vi "翻译助手.vi"() -> ()   [LabVIEW 2014]
uses:
  <vilib>/httpClient/LabVIEWHTTPClient.lvlib
  <vilib>/addons/JSON API/JSON Value/JSON Value.lvclass
  <vilib>/addons/JSON API/JSON Scalar/JSON Scalar.lvclass
panel:
  in  "确定按钮":bool
  in  "目标语言":u16(ring) items=["自动检测", "中文", "英文", "日文", "俄文", "文言文", "粤语", "繁体中文"]
  in  "源语言":u16(ring) items=["自动检测", "中文", "英文", "日文", "俄文", "文言文", "粤语", "繁体中文"]
  out "结果显示":string
  in  "输入文本":string
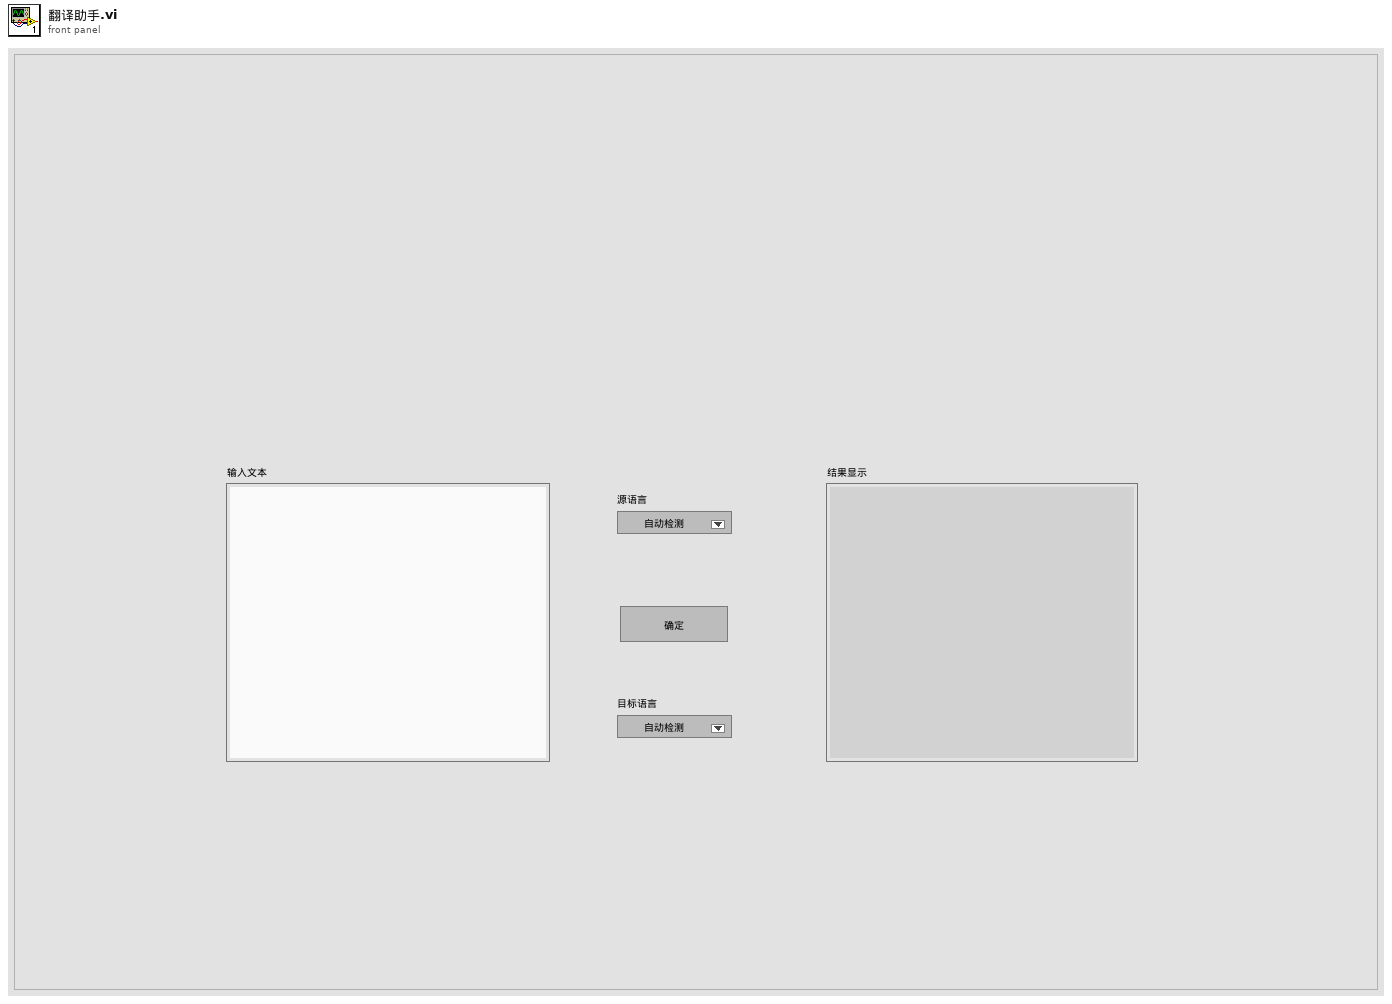
[diagram p1: front panel]
types:
  T1 = typedef "LabVIEWHTTPClient.lvlib/ClientHandle.ctl" = refnum<k1>
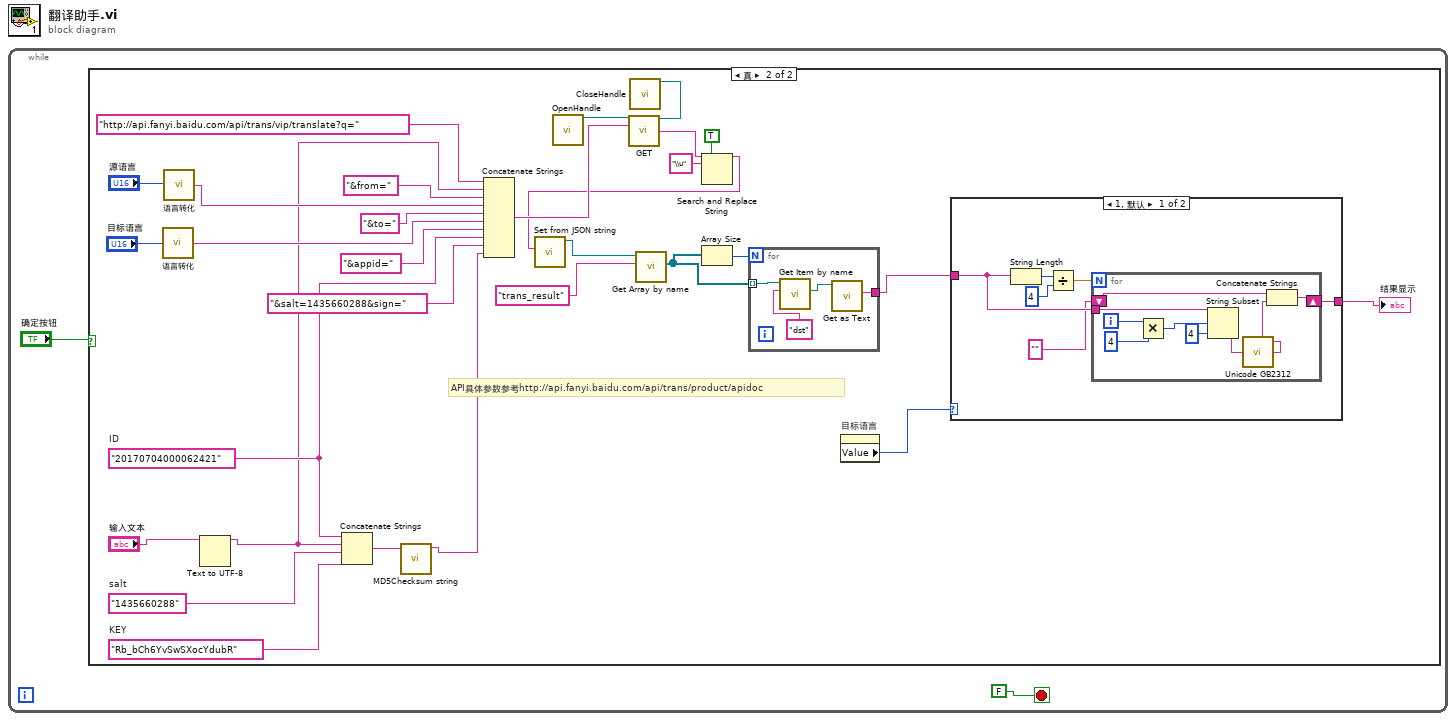
[diagram p0: block diagram]
diagram:
  n1 = while {
    stop <- FALSE stop-if-true
    n2 = case shown="真" "确定按钮" {
      frame False {
      }
      frame True {
        w32 = "1435660288"  # salt
        w31 = "Rb_bCh6YvSwSXocYdubR"  # KEY
        w22 = "20170704000062421"  # ID
        # "API具体参数参考http://api.fanyi.baidu.com/api/trans/product/apidoc"
        n3 = call "语言转化.vi"("选择"="目标语言") -> ("语言"=w24:string)
        n4 = call "语言转化.vi"("选择"="源语言") -> ("语言"=w25:string)
        n5 = Text to UTF-8(11:"输入文本") -> (3:w12:string)  [unwired: 2 in, 1 out]
        n6 = Concatenate Strings(w22, w12, w32, w31) -> (w4:string)
        n7 = call "MD5Checksum string.vi"("Message String"=w4) -> ("MD5 message-digest"=w3:string)  [unwired: 10 in]
        n8 = Concatenate Strings("http://api.fanyi.baidu.com/api/trans/vip/translate?q=", w12, "&from=" ("字符串"), w25, "&to=" ("字符串"), w24, "&appid=", w22, "&salt=1435660288&sign=", w3) -> (w14:string)
        n9 = call <vilib>:"OpenHandle.vi"() -> ("client handle out"=w20:T1)  [unwired: 14 in, 1 out]
        n10 = call <vilib>:"GET.vi"("client handle"=w20, "url"=w14) -> ("client handle out"=w19:T1, "body"=w11:string)  [unwired: 10 in, 2 out]
        n11 = call <vilib>:"CloseHandle.vi"("client handle"=w19) -> ()  [unwired: 14 in, 1 out]
        n12 = Search and Replace String(replace all?=TRUE ("替换全部？(F)"), input string=w11, search string="\\u" ("搜索字符串")) -> (result string=w9:string)  [unwired: 5 in, 3 out]
        n13 = call <vilib>:"Set from JSON string.vi"("JSON stream"=w9) -> ("JSON Value out"=w17:refnum<class "JSON Value.lvclass">)  [unwired: 8 in, 2 out]
        n14 = call <vilib>:"Get Array by name.vi"("name"="trans_result", "JSON Value In"=w17) -> ("Array"=w15:refnum<class "JSON Value.lvclass">[])  [unwired: 6 in, 3 out]
        n15 = Array Size(array=w15) -> (size(s)=w16:i32)
        n16 = for {
          N: w16 -> [_]
          tunnel: w15 -> [w51] mode=indexing
          tunnel: [w49] -> w6
          n17 = call-dynamic "Get Item by name.vi"("name"="dst", "JSON Value In"=w51) -> ("Value"=w50:refnum<class "JSON Value.lvclass">)  [unwired: 6 in, 3 out]
          n18 = call <vilib>:"Get as Text.vi"("JSON Scalar in"=w50) -> ("LabVIEW Text"=w49:string)  [unwired: 8 in, 2 out]
        }
        n19 = property on="目标语言" class="Ring (严格)"() -> ("Value"=w7:u16)  [unwired: 2 in, 2 out]
        n20 = case shown="1, 默认" w7 {
          tunnel: w6 -> [w35 w48]
          tunnel: [w34 w48] -> w5
          frame 1, Default {
            n21 = String Length(string=w35) -> (length=w37:i32)
            n22 = Divide(x=w37, y=4) -> (x/y=w38:dbl)
            n23 = for {
              N: w38 -> [_]
              tunnel: w35 -> [w46]
              shift-right: [w41] -> w34
              shift-left: "" -> [w40]
              i -> [w44]
              n24 = Multiply(x=w44, y=4) -> (x*y=w45:i32)
              n25 = String Subset(string=w46, offset (0)=w45, length (rest)=4 ("长度（剩余）")) -> (substring=w42:string)
              n26 = call "Unicode GB2312.vi"("十六进制源码（不带0x标记）"=w42) -> ("转换后的编码"=w39:string)  [unwired: 14 in]
              n27 = Concatenate Strings(w40, w39) -> (w41:string)
            }
          }
          frame 2 {
          }
        }
        "结果显示" <- w5
      }
    }
  }
